vi "UDP.vi"(1 "error in (no error)":errorcluster) -> (0 "error out":errorcluster)   [LabVIEW 2017]
uses:
  Global.vi
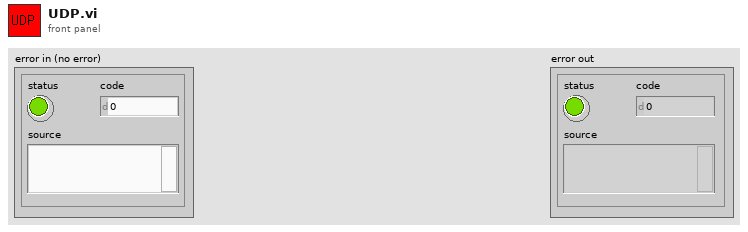
[diagram p1: front panel]
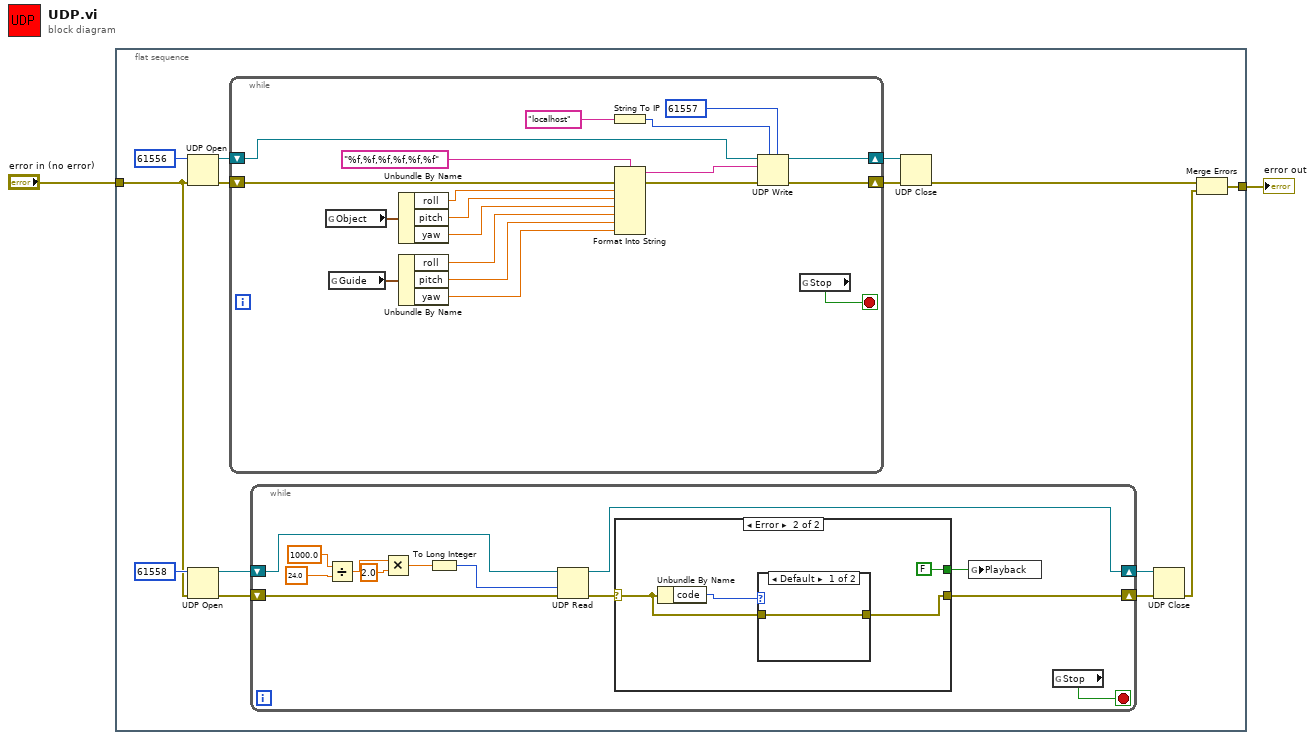
[diagram p0: block diagram]
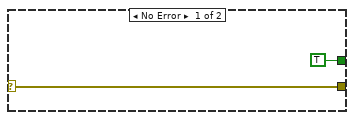
[diagram p2: hidden frame]
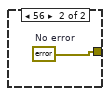
[diagram p3: hidden frame]
diagram:
  n1 = flat-sequence {
    tunnel: "error in (no error)" -> [w8]
    tunnel: [w4] -> w1
    frame #0 {
      n2 = UDP Open(8:w8, 11:u16 61556 ("port")) -> (port=w12:refnum<k16>, 0:w13:errorcluster)  [unwired: 3 in, 1 out]
      n3 = UDP Open(8:w8, 11:u16 61558 ("port")) -> (port=w10:refnum<k16>, 0:w9:errorcluster)  [unwired: 3 in, 1 out]
      n4 = while {
        shift-right: [w56] -> w16
        shift-left: w12 -> [w43]
        shift-right: [w55] -> w15
        shift-left: w13 -> [w42]
        stop <- w50 stop-if-true
        n5 = global read "Global.vi" "Object"() -> (w44:cluster{"roll":dbl, "pitch":dbl, "yaw":dbl})
        n6 = global read "Global.vi" "Guide"() -> (w41:cluster{"roll":dbl, "pitch":dbl, "yaw":dbl})
        n7 = Unbundle By Name(w44) -> ("roll"=w54:dbl, "pitch"=w53:dbl, "yaw"=w52:dbl)
        n8 = Unbundle By Name(w41) -> ("roll"=w40:dbl, "pitch"=w39:dbl, "yaw"=w38:dbl)
        n9 = String To IP(1:"localhost" ("name")) -> (0:w47:u32)
        n10 = Format Into String(format string="%f,%f,%f,%f,%f,%f", error in=w42, w54, w53, w52, w40, w39, w38) -> (resulting string=w45:string, error out=w51:errorcluster)  [unwired: 1 in]
        n11 = UDP Write(address=w47, port or service name=u16 61557, connection ID=w43, data in=w45, 8:w51) -> (error out=w55:errorcluster, 3:w56:refnum<k16>)  [unwired: 1 in]
        n12 = global read "Global.vi" "Stop"() -> (w50:bool)
      }
      n13 = while {
        shift-right: [w26] -> w7
        shift-left: w10 -> [w28]
        shift-right: [w17] -> w3
        shift-left: w9 -> [w29]
        stop <- w27 stop-if-true
        n14 = Divide(x=1000.0, y=24.0) -> (x/y=w23:dbl)
        n15 = Multiply(x=w23, y=2.0) -> (x*y=w21:dbl)
        n16 = To Long Integer(number=w21) -> (32bit integer=w20:i32)
        n17 = UDP Read(connection ID=w28, timeout ms (25000)=w20, 8:w29) -> (error out=w19:errorcluster, 3:w26:refnum<k16>)  [unwired: 1 in, 3 out]
        n18 = case shown="Error" w19 {
          selector: w19 -> [w30 w33]
          tunnel: [TRUE ("Playback") FALSE ("Playback")] -> w18
          tunnel: [w30 w34] -> w17
          frame No Error {
          }
          frame Error {
            n19 = Unbundle By Name(w33) -> ("code"=w32:i32)
            n20 = case shown="Default" w32 {
              tunnel: w33 -> [w36 _]
              tunnel: [w36 w37] -> w34
              frame Default {
              }
              frame 56 {
                w37 = errorcluster {"status"=FALSE, "code"=0, "source"=""}  # No error
              }
            }
          }
        }
        n21 = global write "Global.vi" "Playback"(w18) -> ()
        n22 = global read "Global.vi" "Stop"() -> (w27:bool)
      }
      n23 = UDP Close(connection ID=w16, 8:w15) -> (error out=w6:errorcluster)  [unwired: 1 out]
      n24 = UDP Close(connection ID=w7, 8:w3) -> (error out=w5:errorcluster)  [unwired: 1 out]
      n25 = Merge Errors(w6, w5) -> (w4:errorcluster)
    }
  }
  "error out" <- w1
